vi "VisaScan.vi"(8 "errin":errorcluster) -> (0 "errout":errorcluster caption="error out", 1 "NextStep":T2=enum."Scan", 3 "VISA OUT":T1)   [LabVIEW 2020]
uses:
  OP500Z8_state.ctl
  <vilib>/Instr/_visa.llb/VISA Find Search Mode.ctl
  C:/Users/elhajj/OneDrive - FORSEE POWER/Bureau/Support banc de test/Ligne ZENPLUS/Code LabVIEW/CODE/02 SLIM ZEN WS 500/SubVi/FGV.ctl
  c81239b7-4444-44a5-8c00-ba4ac2918693.vi
  VG/VG_EquipementsNeeded.vi
  <instrlib>/IT6000C/IT6000C.lvlib
panel:
  out "Refaire":bool
  in  "VISA IN":T1
  out "Equipements OK ?":bool[](array[boolean])
  out "liste trouvée":string[](array[string])
  # "ITECH\n\nST5520\n\nTENMA\n\nBT5564"
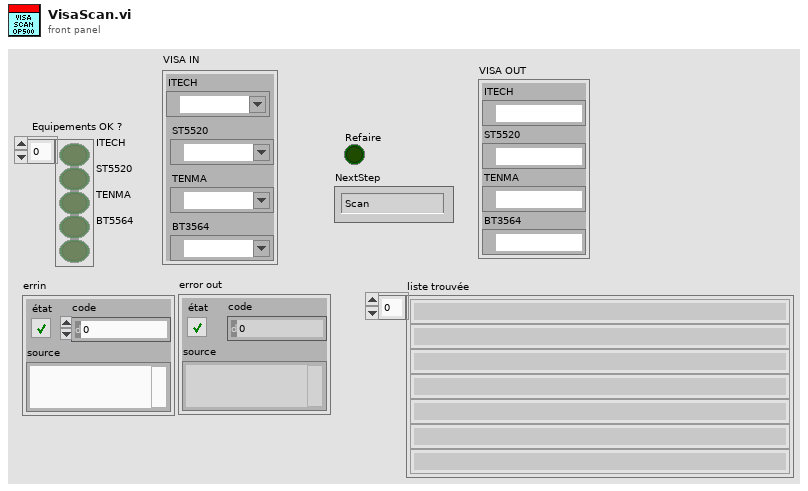
[diagram p1: front panel]
types:
  T1 = cluster{"ITECH":refnum<visa-resource-name>, "ST5520":refnum<visa-resource-name>, "TENMA":refnum<visa-resource-name>, "BT3564":refnum<visa-resource-name>}
  T2 = typedef "OP500Z8_state.ctl" = enum16{"Null", "Demarrage", "Init", "Scan", "Montage", "OCV", "Iso", "DataDyn", "Demontage", "Crash", "Next", "GoDCIR", "DCIR", "EXIT", "LogErr", "DTC"}
  T3 = typedef "VISA Find Search Mode.ctl" = u32
  T4 = typedef "FGV.ctl" = enum16{"GET", "SET", "RAZ"}
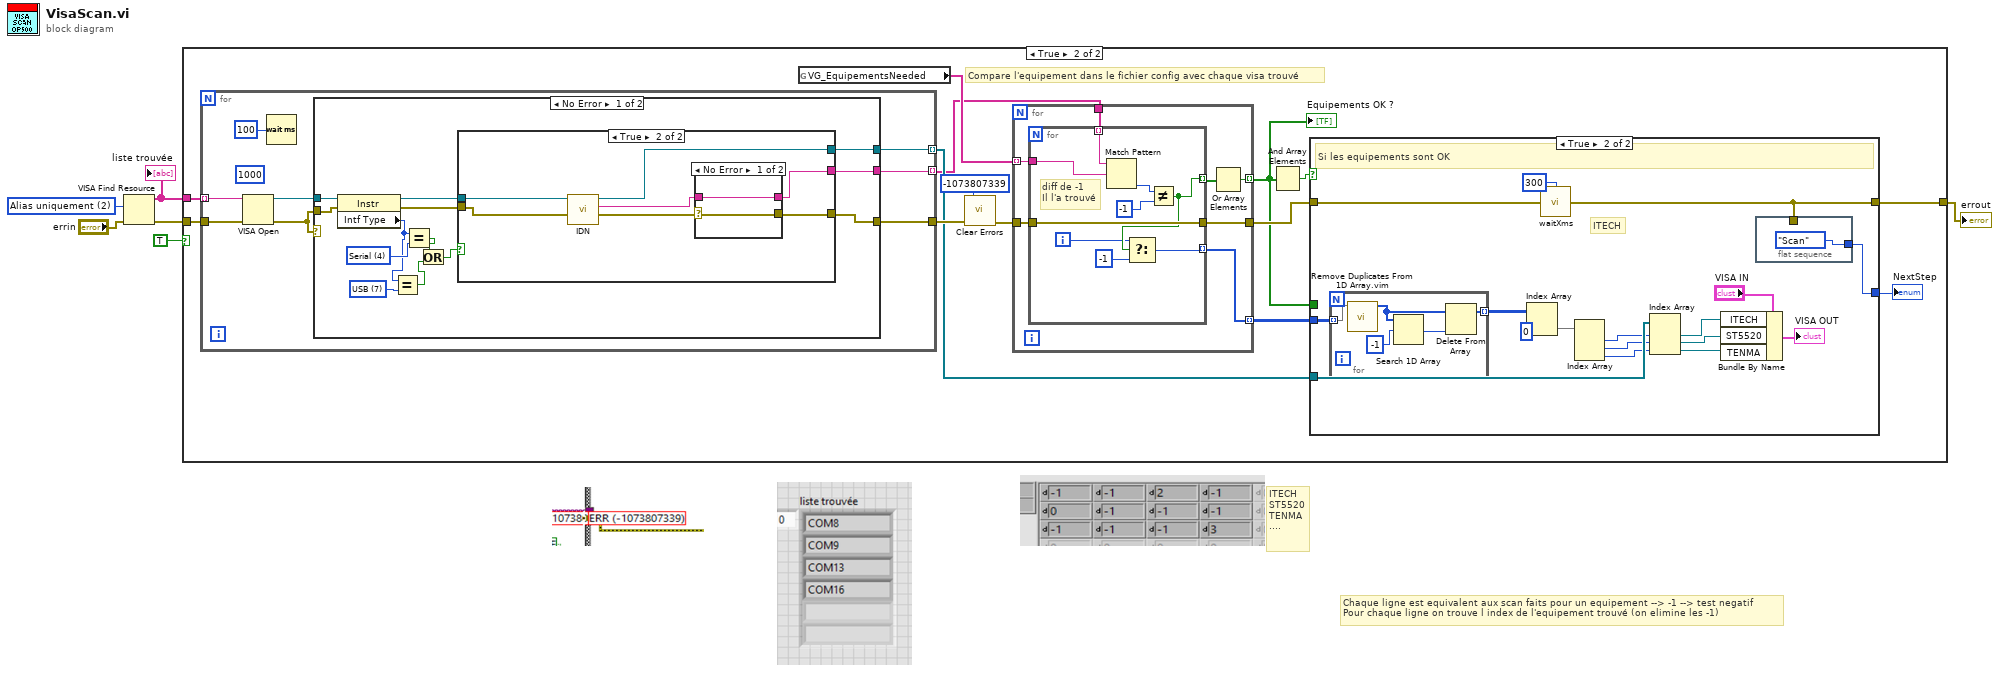
[diagram p0: block diagram]
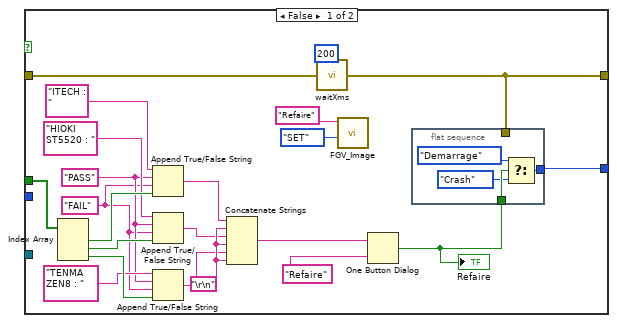
[diagram p3: hidden frame]
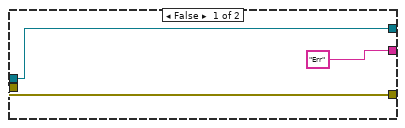
[diagram p4: hidden frame]
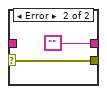
[diagram p5: hidden frame]
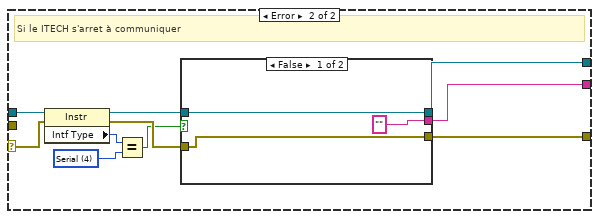
[diagram p6: hidden frame]
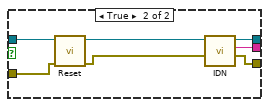
[diagram p7: hidden frame]
diagram:
  w5 = T3 2 items=["Noms canoniques uniquement"=0, "Alias uniquement"=2, "Inclure les alias correspondants"=3, "Inclure tous les alias"=4] ("Search Mode")
  # "ITECH\nST5520\nTENMA\n...."
  # "Chaque ligne est equivalent aux scan faits pour un equipement --> -1 --> test negatif\nPour chaque ligne on trouve l index de l'equipement trouvé (on elimine les -1)"
  n1 = VISA Find Resource(8:"errin", 10:w5) -> (0:w3:errorcluster, 3:w4:string[])  [unwired: 1 in, 1 out]
  "liste trouvée" <- w4
  n2 = case shown="True" TRUE {
    tunnel: w4 -> [_ w21]
    tunnel: w3 -> [w7 w20]
    tunnel: [w7 w14] -> w2
    frame False {
    }
    frame True {
      # "Compare l'equipement dans le fichier config avec chaque visa trouvé"
      n3 = for {
        tunnel: w21 -> [w90] mode=indexing
        tunnel: [w94] -> w10 mode=indexing
        tunnel: w20 -> [w89]
        tunnel: [w92] -> w18
        tunnel: [w91] -> w11 mode=indexing
        (unwired) u32 1000 ("timeout (10sec)")
        n4 = VISA Open(error in (no error)=w89, VISA resource name=w90) -> (VISA resource name=w88:refnum<visa-resource-name>, error out=w87:errorcluster)  [unwired: 3 in]
        n5 = Wait (ms)(milliseconds to wait=u32 100 ("attente (ms)")) -> ()  [unwired: 1 out]
        n6 = case shown="No Error" w87 {
          selector: w87 -> [_ w124]
          tunnel: w87 -> [w107 _]
          tunnel: w88 -> [w106 w127]
          tunnel: [w102 w130] -> w94
          tunnel: [w101 w129] -> w92
          tunnel: [w100 w131] -> w91
          frame No Error {
            w99 = u16 7 items=["GPIB"=1, "VXI"=2, "GPIB-VXI"=3, "Serial"=4, "PXI"=5, "TCPIP"=6, "USB"=7, "FireWire"=9] ("Interface Information:Interface Type")
            w105 = u16 4 items=["GPIB"=1, "VXI"=2, "GPIB-VXI"=3, "Serial"=4, "PXI"=5, "TCPIP"=6, "USB"=7, "FireWire"=9] ("Interface Information:Interface Type")
            n7 = property class="Instr"(reference=w106, error in=w107) -> (reference out=w103:refnum<visa-resource-name>, error out=w104:errorcluster, "Intf Type"=w95:u16)
            n8 = Equal?(x=w95, y=w99) -> (x = y?=w96:bool)
            n9 = Equal?(x=w95, y=w105) -> (x = y?=w97:bool)
            n10 = Or(x=w97, y=w96) -> (x .or. y?=w98:bool)
            n11 = case shown="True" w98 {
              tunnel: w104 -> [w110 w111]
              tunnel: w103 -> [w109 w112]
              tunnel: ["Err" ("read buffer") w117] -> w102
              tunnel: [w110 w116] -> w101
              tunnel: [w109 w114] -> w100
              frame False {
              }
              frame True {
                n12 = call "IDN"("errin"=w111, "VISAin"=w112) -> ("error out"=w113:errorcluster, "ID"=w115:string, "VISA Refnum out"=w114:refnum<visa-resource-name>)  [unwired: 5 in]
                n13 = case shown="No Error" w113 {
                  selector: w113 -> [w118 w120]
                  tunnel: w115 -> [w119 _]
                  tunnel: [w119 ""] -> w117
                  tunnel: [w118 w120] -> w116
                  frame No Error {
                  }
                  frame Error {
                  }
                }
              }
            }
          }
          frame Error {
            w128 = u16 4 items=["GPIB"=1, "VXI"=2, "GPIB-VXI"=3, "Serial"=4, "PXI"=5, "TCPIP"=6, "USB"=7, "FireWire"=9] ("Interface Information:Interface Type")
            # "Si le ITECH s'arret à communiquer"
            n14 = property class="Instr"(reference=w127, error in=w124) -> (reference out=w126:refnum<visa-resource-name>, error out=w125:errorcluster, "Intf Type"=w123:u16)
            n15 = Equal?(x=w123, y=w128) -> (x = y?=w122:bool)
            n16 = case shown="False" w122 {
              tunnel: [w133 w141] -> w131
              tunnel: ["" ("ID") w140] -> w130
              tunnel: [w134 w139] -> w129
              tunnel: w126 -> [w133 w138]
              tunnel: w125 -> [w134 w137]
              frame False {
              }
              frame True {
                n17 = call <instrlib>:"Reset.vi"("error in (no error)"=w137, "VISA resource name"=w138) -> ("error out"=w136:errorcluster, "VISA resource name out"=w135:refnum<visa-resource-name>)  [unwired: 8 in]
                n18 = call "IDN"("errin"=w136, "VISAin"=w135) -> ("error out"=w139:errorcluster, "ID"=w140:string, "VISA Refnum out"=w141:refnum<visa-resource-name>)  [unwired: 5 in]
              }
            }
          }
        }
      }
      n19 = global read "VG_EquipementsNeeded.vi" "VG_EquipementsNeeded"() -> (w16:string[])
      n20 = call <vilib>:"Clear Errors.vi"("error in (no error)"=w18, "specific error code to clear (0: all)"=-1073807339) -> ("error out"=w17:errorcluster)  [unwired: 4 in, 1 out]
      n21 = for {
        tunnel: [w72] -> w12 mode=indexing
        tunnel: w17 -> [w77]
        tunnel: [w76] -> w15
        tunnel: w10 -> [w75]
        tunnel: w16 -> [w74] mode=indexing
        tunnel: [w71] -> w8 mode=indexing
        n22 = for {
          tunnel: w77 -> [w86]
          tunnel: [w86] -> w76
          tunnel: [w81] -> w73 mode=indexing
          tunnel: w75 -> [w83] mode=indexing
          tunnel: w74 -> [w82]
          tunnel: [w78] -> w71 mode=indexing
          i -> [w80]
          # "diff de -1\nIl l'a trouvé"
          n23 = Match Pattern(string=w83, regular expression=w82) -> (offset past match=w84:i32)  [unwired: 1 in, 3 out]
          n24 = Not Equal?(x=w84, y=-1) -> (x != y?=w81:bool)
          n25 = Select(t=w80, s=w81, f=-1 ("cas faux")) -> (s? t:f=w78:i32)
        }
        n26 = Or Array Elements(Boolean array=w73) -> (logical OR=w72:bool)
      }
      "Equipements OK ?" <- w12
      n27 = And Array Elements(Boolean array=w12) -> (logical AND=w13:bool)
      n28 = case shown="True" w13 {
        tunnel: w15 -> [w25 w62]
        tunnel: [w24 w60] -> w14
        tunnel: w12 -> [w42 _]
        tunnel: w11 -> [_ w64]
        tunnel: [w22 w61] -> w9
        tunnel: w8 -> [_ w54]
        frame False {
          w33 = "FAIL" ("nom du bouton (\"OK\")")
          w34 = "PASS" ("nom du bouton (\"OK\")")
          w31 = "\r\n"
          n29 = Index Array(array=w42) -> (element #1=w41:bool, element #2=w40:bool, element #3=w39:bool)  [unwired: 3 in]
          n30 = Append True/False String(1:w41, 2:w33, 3:w34, 4:"ITECH : " ("nom du bouton (\"OK\")")) -> (0:w35:string)
          n31 = Append True/False String(1:w40, 2:w33, 3:w34, 4:"HIOKI ST5520 : " ("nom du bouton (\"OK\")")) -> (0:w30:string)
          n32 = Append True/False String(1:w39, 2:w33, 3:w34, 4:"TENMA ZEN8 : " ("nom du bouton (\"OK\")")) -> (0:w29:string)
          n33 = Concatenate Strings(w35, w31, w30, w31, w29, w31) -> (w32:string)
          n34 = call <userlib>:"waitXms.vi"("attente (ms)"=u32 200, "errin"=w25) -> ("errout"=w24:errorcluster)  [unwired: 13 in]
          n35 = call "FGV_Image.vi"("Énum"=FGV."SET", "IN"="Refaire") -> ()  [unwired: 9 in, 1 out]
          n36 = One Button Dialog(message=w32, button name ("OK")="Refaire" ("nom du bouton (\"OK\")")) -> (true=w23:bool)
          "Refaire" <- w23
          n37 = flat-sequence {
            tunnel: w24 -> [_]
            tunnel: w23 -> [w47]
            tunnel: [w44] -> w22
            frame #0 {
              n38 = Select(t=OP500Z8_state."Demarrage" ("Énum"), s=w47, f=OP500Z8_state."Crash" ("cas faux")) -> (s? t:f=w44:T2)
            }
          }
        }
        frame True {
          # "ITECH"
          # "Si les equipements sont OK"
          n39 = for {
            tunnel: w54 -> [w69] mode=indexing
            tunnel: [w66] -> w53 mode=indexing
            n40 = call "Remove Duplicates From 1D Array.vim"("array"=w69) -> ("array with duplicates removed"=w67:i32[])  [unwired: 10 in]
            n41 = Search 1D Array(1D array=w67, element=-1 ("élément")) -> (index of element=w65:i32)  [unwired: 1 in]
            n42 = Delete From Array(array=w67, index=w65) -> (array with subset deleted=w66:i32[])  [unwired: 1 in, 1 out]
          }
          n43 = Index Array(array=w53, index (col)=0 ("indice désactivé (col)")) -> (element=w51:i32[])  [unwired: 1 in]
          n44 = call <userlib>:"waitXms.vi"("attente (ms)"=u32 300, "errin"=w62) -> ("errout"=w60:errorcluster)  [unwired: 13 in]
          n45 = Index Array(array=w51) -> (element #1=w50:i32, element #2=w49:i32, element #3=w48:i32)  [unwired: 3 in]
          n46 = Index Array(array=w64, index #1=w50, index #2=w49, index #3=w48) -> (element #1=w58:refnum<visa-resource-name>, element #2=w57:refnum<visa-resource-name>, element #3=w56:refnum<visa-resource-name>)
          n47 = Bundle By Name(cluster="VISA IN", "ITECH"=w58, "ST5520"=w57, "TENMA"=w56) -> (→"VISA OUT":T1)
          n48 = flat-sequence {
            tunnel: [OP500Z8_state."Scan" ("Énum")] -> w61
            tunnel: w60 -> [_]
            frame #0 {
            }
          }
        }
      }
      "NextStep" <- w9
    }
  }
  "errout" <- w2
